vi "str_dis.vi"() -> ()   [LabVIEW 2019]
uses:
  <vilib>/Platform/TimedLoop/XDataNode/timing_clust.ctl
  <vilib>/Platform/TimedLoop/XDataNode/nitl_modes.ctl
  <vilib>/Platform/TimedLoop/XDataNode/wakeup.ctl
  <vilib>/myRIO/Instrument Drivers/Onboard IO/UART/typedef/VISA Configuration.ctl
  <vilib>/Instr/_visa.llb/VISA Configure Serial Port (Instr).vi
  <vilib>/Platform/TimedLoop/XDataNode/XDataNode.xnode
  <vilib>/myRIO/Express VI/Onboard IO/UART/UART Express VI.xnode
  <vilib>/myRIO/Instrument Drivers/Onboard IO/UART/UART.lvlib
  <vilib>/Platform/TimedLoop/XDataNode/XDNodeRunTimeDep.lvlib
panel:
  out "숫자형":i32
  out "error out 2":errorcluster caption="에러 출력"
  in  "error in (no error) 2":errorcluster caption="에러 입력(에러 없음)"
  in  "정지 2":bool
  out "숫자형 2":i32
  out "Characters Read":string
  out "error out":errorcluster caption="에러 출력"
  in  "error in (no error)":errorcluster caption="에러 입력(에러 없음)"
  in  "정지":bool
  out "2번":string
  out "3번":string
  out "1번":string
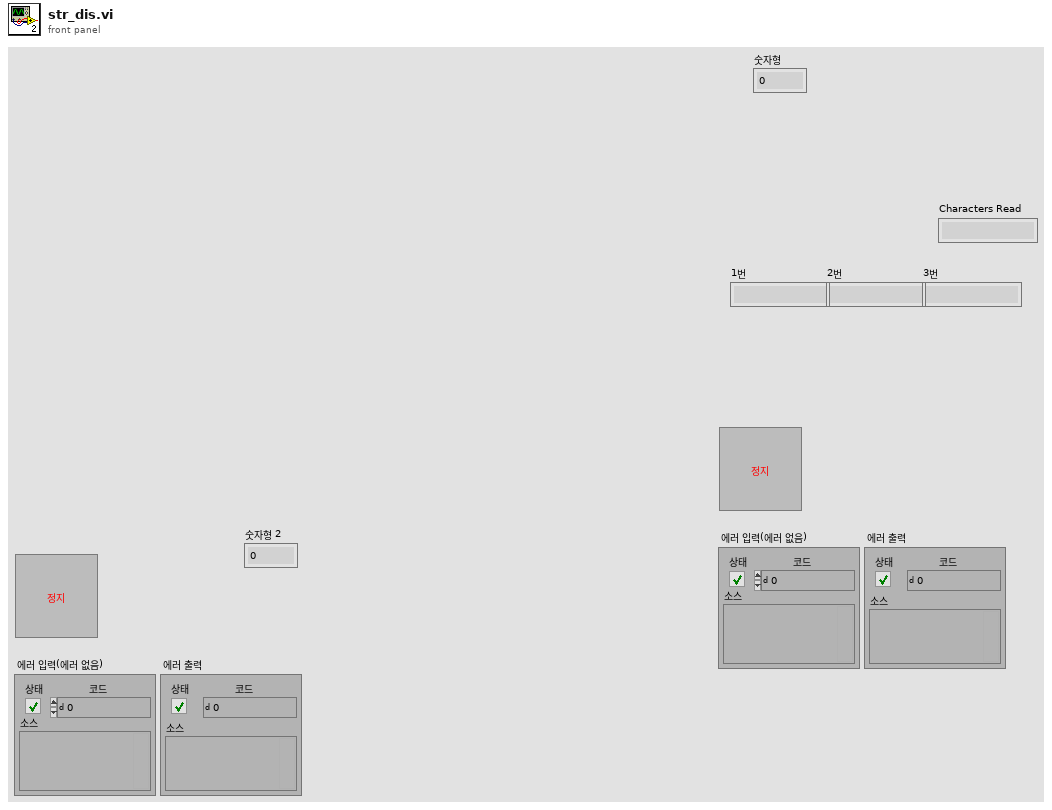
[diagram p1: front panel]
types:
  T1 = typedef "UART.lvlib/VISA Configuration.ctl" = cluster{"baud rate (9600)":u32, "data bits (8)":u16, "parity (0:none)":enum16{"None", "Odd", "Even", "Mark", "Space"}, "stop bits (10: 1 bit)":u16, "flow control (0:none)":u16, "termination char\n(0xA = '\\n' = LF) ":u8, "Enable Termination\nChar (T)":bool, "timeout (10sec)":u32}
  T2 = typedef "XDNodeRunTimeDep.lvlib/timing_clust.ctl" = cluster{"Expected End [f-1]":u64, "Actual End [f-1]":u64, "Finished Late? [f-1]":bool, "Expected End [i-1]":u64, "Actual End [i-1]":u64, "Finished Late? [i-1]":bool, "Expected Start [i]":u64, "Actual Start [i]":u64, "Expected Start [f]":u64, "Actual Start [f]":u64, "Source Name":string, "Structure Name":string, "Period":i64, "Deadline":i64, "Offset":i64, "Start":i64, "Priority":i32, "Timeout":i32, "Mode":T3, "Wakeup Reason":T4, "Error":errorcluster, "Source Type":string, "Secondary Source Type":string, "Global End Time":u64, "Global Start Time":u64, "Frame Duration":u64, "Iteration Duration":u64, "Assigned CPU":i32, "I/O Scan Engine Mode":u32}
  T3 = typedef "XDNodeRunTimeDep.lvlib/nitl_modes.ctl" = enum32{"No Change", "Process missed periods, maintain original phase", "Discard missed periods, maintain original phase", "Process missed periods, ignore original phase", "Discard missed periods, ignore original phase"}
  T4 = typedef "XDNodeRunTimeDep.lvlib/wakeup.ctl" = enum32{"Normal", "Aborted", "Asynchronous wakeup", "Timing source error", "Timed loop error", "Timeout"}
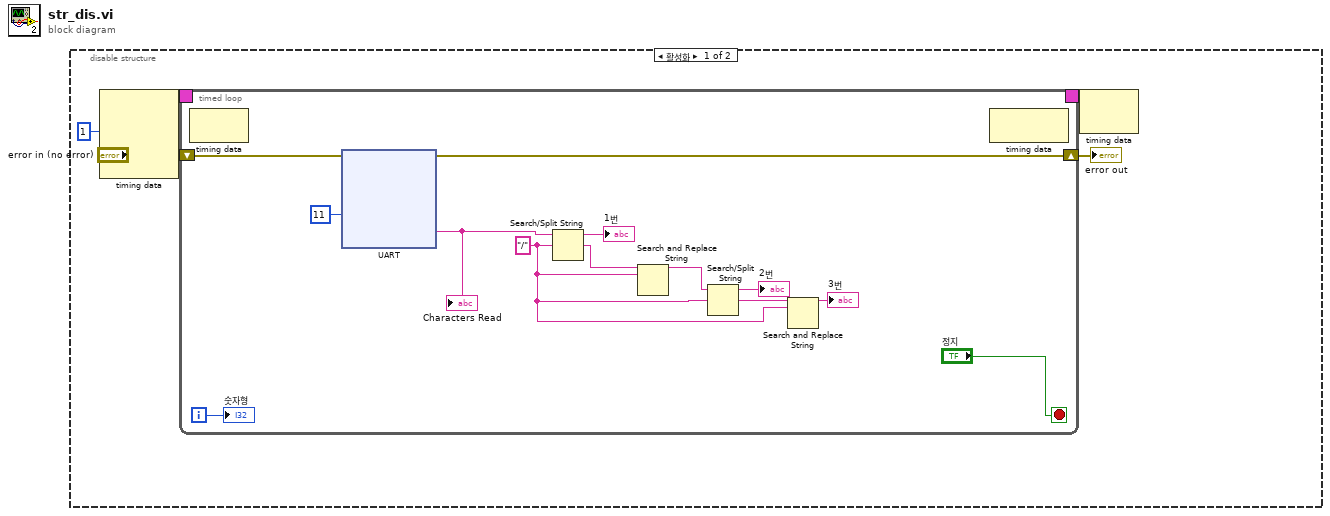
[diagram p0: block diagram]
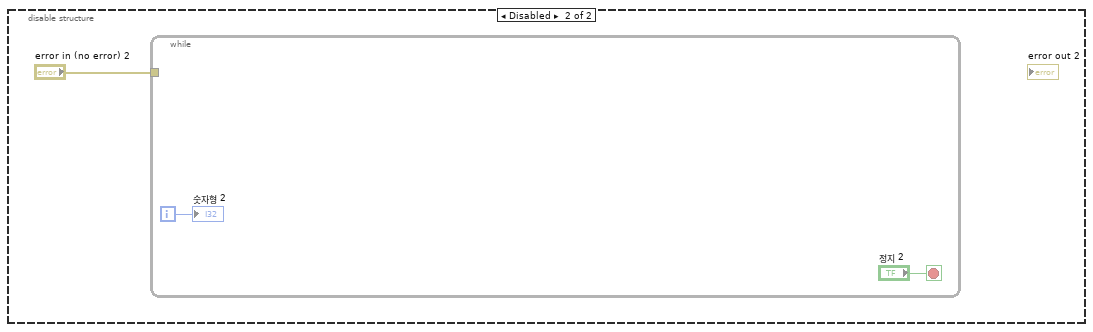
[diagram p2: hidden frame]
diagram:
  n1 = disable-structure shown="활성화" {
    frame Enabled {
      n2 = node-c288(i64 1 ("주기")) -> (w3:T2)  [unwired: 3 in]
      n3 = timed-loop {
        timing: w3 -> [_]
        timing-out: [_] -> w2
        shift-right: [w17] -> w4
        shift-left: "error in (no error)" -> [w18]
        i -> [w7]
        stop <- "정지" stop-if-true
        w10 = "/" ("검색 문자열/문자 (-)")
        n4 = node-c288() -> ()  [unwired: 1 in, 1 out]
        n5 = xnode "UART"("Character Count"=u32 11, "error in (no error)"=w18) -> ("Characters Read"=w9:string, "error out"=w17:errorcluster)
        "Characters Read" <- w9
        n6 = Search/Split String(string=w9, search string/char (-)=w10) -> (substring before match=→"1번":string, match + rest of string=w11:string)  [unwired: 2 out]
        n7 = Search and Replace String(input string=w11, search string=w10) -> (result string=w13:string)  [unwired: 1 in, 8 out]
        n8 = Search/Split String(string=w13, search string/char (-)=w10) -> (substring before match=→"2번":string, match + rest of string=w12:string)  [unwired: 2 out]
        n9 = Search and Replace String(input string=w12, search string=w10) -> (result string=→"3번":string)  [unwired: 1 in, 8 out]
        n10 = node-c288() -> ()  [unwired: 1 in, 1 out]
        "숫자형" <- w7
      }
      "error out" <- w4
      n11 = node-c288(w2) -> ()  [unwired: 1 out]
    }
    frame Disabled {
      n12 = while {
        tunnel: "error in (no error) 2" -> [_]
        i -> [w42]
        stop <- "정지 2" stop-if-true
        "숫자형 2" <- w42
      }
    }
  }
